vi "Unregister Feeds Containing Search String.vi"(8 "error in (no error)":errorcluster, 11 "search string":string) -> (0 "error out":errorcluster)   [LabVIEW 2014]
doc: "Unregisters any previously registered feeds with a feed name containing the specified search string"
uses:
  <vilib>/National Instruments/NIPM API (Beta)/NIPM_API.lvlib
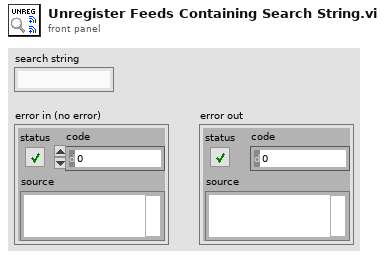
[diagram p1: front panel]
types:
  T1 = typedef "NIPM_API.lvlib/feed.ctl" = cluster{"Name":string, "URI":string}
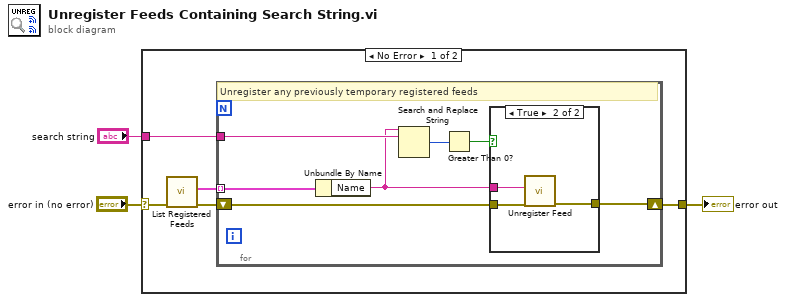
[diagram p0: block diagram]
diagram:
  n1 = case shown="No Error" "error in (no error)" {
    selector: "error in (no error)" -> [w4 w20]
    tunnel: [w8 w20] -> w3
    tunnel: "search string" -> [w6 _]
    frame No Error {
      n2 = call <vilib>:"List Registered Feeds.vi"("error in"=w4) -> ("error out"=w7:errorcluster, "registered feeds"=w5:T1[])  [unwired: 9 in]
      n3 = for {
        tunnel: w5 -> [w15] mode=indexing
        tunnel: w6 -> [w14]
        shift-right: [w10] -> w8
        shift-left: w7 -> [w11]
        # "Unregister any previously temporary registered feeds"
        n4 = Unbundle By Name(w15) -> ("Name"=w12:string)
        n5 = Search and Replace String(input string=w12, search string=w14) -> (number of replacements=w13:i32)  [unwired: 6 in, 3 out]
        n6 = Greater Than 0?(x=w13) -> (x > 0?=w9:bool)
        n7 = case shown="True" w9 {
          tunnel: w12 -> [_ w19]
          tunnel: w11 -> [w16 w18]
          tunnel: [w16 w17] -> w10
          frame False {
          }
          frame True {
            n8 = call <vilib>:"Unregister Feed.vi"("error in"=w18, "feed name"=w19) -> ("error out"=w17:errorcluster)  [unwired: 8 in, 1 out]
          }
        }
      }
    }
    frame Error {
    }
  }
  "error out" <- w3
